vi "HRM-process-calculate_heartrate.vi"(8 "error in (no error)":errorcluster, 11 "Process data":T1={"Raw collected data"={"t0"=timestamp(0 s since 1904-01-01), "dt"=1.0, "Y"=[]}, "filtered data"={"t0"=timestamp(0 s since 1904-01-01), "dt"=1.0, "Y"=[]}, "Heartrate"=0.0, "Additional Signal to remove [s]"=0, "samples [s]"=10, "Pulse settings"={"Manual?"=FALSE, "Top"=0.0, "Bottom"=0.0}, "User Events"={"Additional Signal to remove [s]"=refnum, "samples [s]"=refnum, "Heart Rate"=refnum, "Raw collected data"=refnum, "Filtered data"=refnum, "Raw Data"=refnum, "stop"=refnum, "Status Feedback"=refnum, "pause AQN"=refnum, "Clear wf Data"=refnum, "Pulse settings"=refnum}}) -> (0 "error out":errorcluster, 3 "Process data ouy":T1={"Raw collected data"={"t0"=timestamp(0 s since 1904-01-01), "dt"=1.0, "Y"=[]}, "filtered data"={"t0"=timestamp(0 s since 1904-01-01), "dt"=1.0, "Y"=[]}, "Heartrate"=0.0, "Additional Signal to remove [s]"=0, "samples [s]"=10, "Pulse settings"={"Manual?"=FALSE, "Top"=0.0, "Bottom"=0.0}, "User Events"={"Additional Signal to remove [s]"=refnum, "samples [s]"=refnum, "Heart Rate"=refnum, "Raw collected data"=refnum, "Filtered data"=refnum, "Raw Data"=refnum, "stop"=refnum, "Status Feedback"=refnum, "pause AQN"=refnum, "Clear wf Data"=refnum, "Pulse settings"=refnum}})   [LabVIEW 2020]
uses:
  HRM-process-loop_data.ctl
  HRM-process-Pulse settings.ctl
  init/HRM-init-user_events.ctl
  <vilib>/measure/matone.llb/Extract Single Tone Information 1 Chan.vi
  <vilib>/measure/NI_MAPro.lvlib
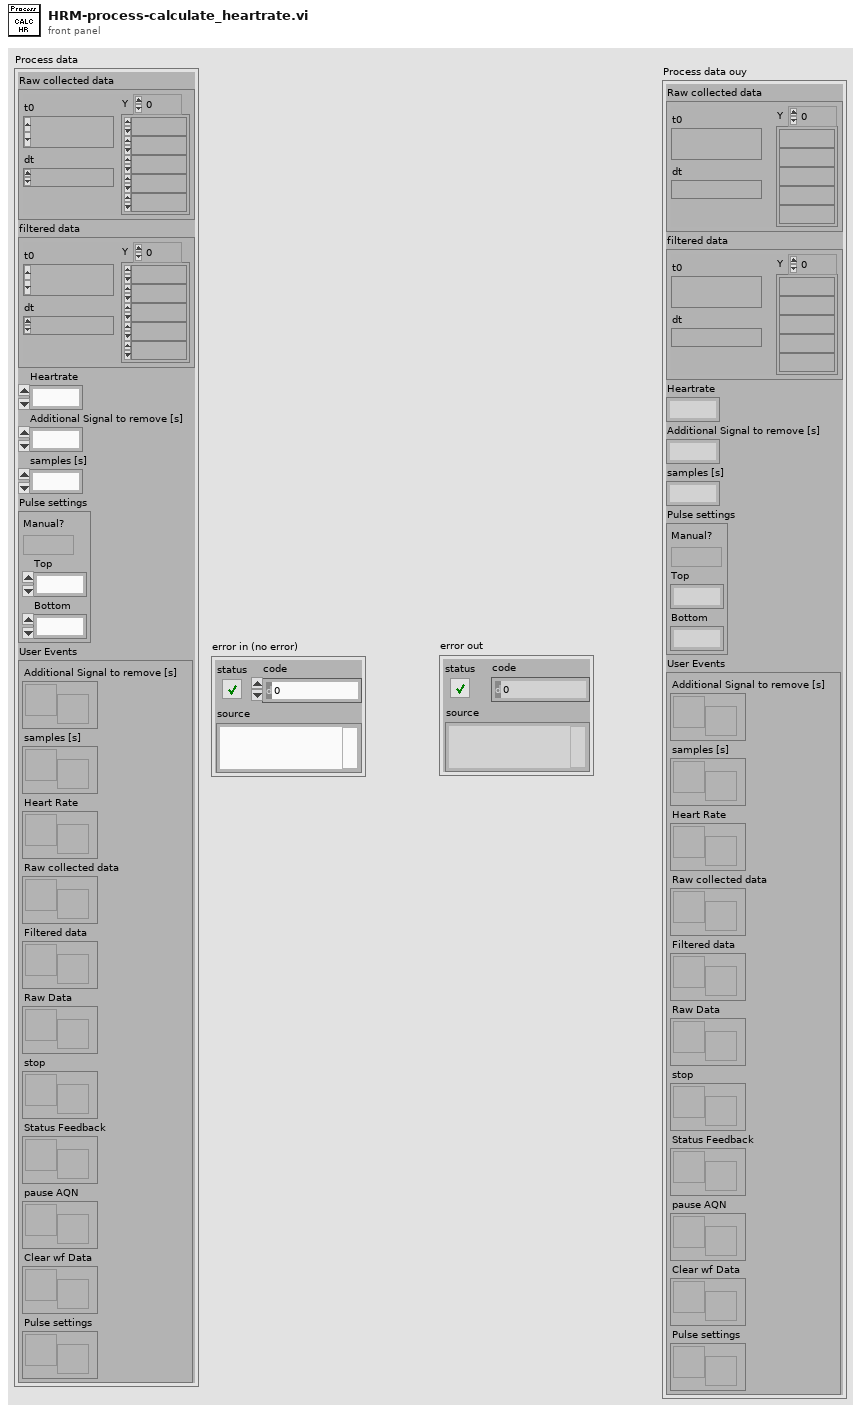
[diagram p1: front panel]
types:
  T1 = typedef "HRM-process-loop_data.ctl" = cluster{"Raw collected data":waveform(dbl), "filtered data":waveform(dbl), "Heartrate":dbl, "Additional Signal to remove [s]":i32, "samples [s]":i32, "Pulse settings":T2, "User Events":T3}
  T2 = typedef "HRM-process-Pulse settings.ctl" = cluster{"Manual?":bool, "Top":dbl, "Bottom":dbl}
  T3 = typedef "HRM-init-user_events.ctl" = cluster{"Additional Signal to remove [s]":refnum<user-event>, "samples [s]":refnum<user-event>, "Heart Rate":refnum<user-event>, "Raw collected data":refnum<user-event>, "Filtered data":refnum<user-event>, "Raw Data":refnum<user-event>, "stop":refnum<user-event>, "Status Feedback":refnum<user-event>, "pause AQN":refnum<user-event>, "Clear wf Data":refnum<user-event>, "Pulse settings":refnum<user-event>}
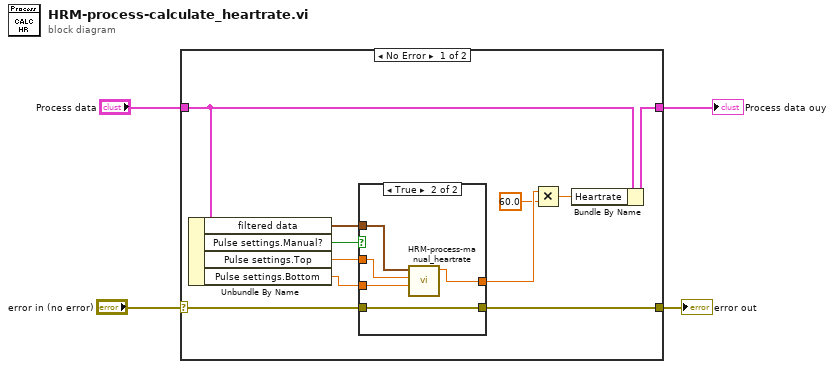
[diagram p0: block diagram]
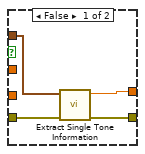
[diagram p2: hidden frame]
diagram:
  n1 = case shown="No Error" "error in (no error)" {
    selector: "error in (no error)" -> [w11 w25]
    tunnel: [w10 w25] -> w3
    tunnel: "Process data" -> [w14 w26]
    tunnel: [w15 w26] -> w1
    frame No Error {
      n2 = Unbundle By Name(w14) -> ("filtered data"=w9:waveform(dbl), "Pulse settings.Manual?"=w7:bool, "Pulse settings.Top"=w6:dbl, "Pulse settings.Bottom"=w5:dbl)
      n3 = case shown="True" w7 {
        tunnel: [w19 w22] -> w13
        tunnel: w11 -> [w18 w24]
        tunnel: [w17 w24] -> w10
        tunnel: w9 -> [w16 w23]
        tunnel: w6 -> [_ w21]
        tunnel: w5 -> [_ w20]
        frame False {
          n4 = call-poly <vilib>:"Extract Single Tone Information.vi"("error in (no error)"=w18, "time signal in"=w16) -> ("error out"=w17:errorcluster, "detected frequency"=w19:dbl)  [unwired: 4 in, 4 out]
        }
        frame True {
          n5 = call "HRM-process-manual_heartrate.vi"("Bottom"=w20, "Top"=w21, "data in"=w23) -> ("Frequency [Hz]"=w22:dbl)  [unwired: 8 in]
        }
      }
      n6 = Multiply(x=w13, y=60.0) -> (x*y=w8:dbl)
      n7 = Bundle By Name(cluster=w14, "Heartrate"=w8) -> (w15:T1)
    }
    frame Error {
    }
  }
  "Process data ouy" <- w1
  "error out" <- w3
